vi "Read Configuration(Variant).vi"(6 "Strict type matching? (F)":bool, 7 "Qualified Name":string, 8 "error in (no error)":errorcluster, 9 "Name (empty: value name)":string, 10 "Default value":variant, 11 "Attribute.Config in":refnum<class "Attribute.Config.lvclass">) -> (0 "error out":errorcluster, 1 "any found?":bool, 2 "Variant":variant, 3 "Attribute.Config out":refnum<class "Attribute.Config.lvclass">, 4 "all found?":bool)   [LabVIEW 2013, in "Attribute.Config.lvclass"]
uses:
  Attribute.Config.lvclass
  Attribute.Config.lvclass/Attribute.Config.ctl
  <vilib>/LabVIEW Open Source Project/Configuration Manager/Manager/ConfigManager.lvclass
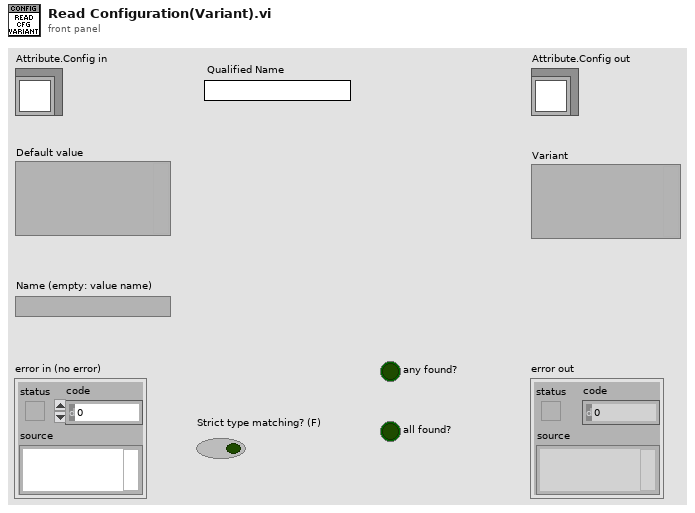
[diagram p1: front panel]
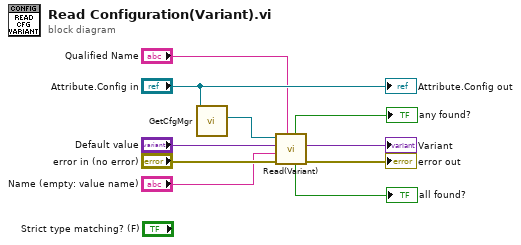
[diagram p0: block diagram]
diagram:
  n1 = call "GetCfgMgr.vi"("Attribute.Config in"="Attribute.Config in") -> ("CfgMgr"=w9:refnum<class "ConfigManager.lvclass">)  [unwired: 9 in, 1 out]
  n2 = call <vilib>:"Read(Variant).vi"("Qualified Name"="Qualified Name", "error in (no error)"="error in (no error)", "Name (empty: type name)"="Name (empty: value name)", "Type"="Default value", "ConfigManager in"=w9) -> ("error out"=→"error out":errorcluster, "value"=→"Variant":variant, "all found?"=→"all found?":bool, "any found?"=→"any found?":bool)  [unwired: 2 in, 1 out]
  "Attribute.Config out" <- "Attribute.Config in"
